vi "Write_Parameter_To_Node_Test.vi"() -> ()   [LabVIEW 2017]
uses:
  Classes/ADCP.lvclass
panel:
  in  "ADCP in":refnum<class "ADCP.lvclass">
  in  "Write Parameter":bool
  in  "Parameter value":string
  in  "Parameter name":string(combo)
  in  "Stop Application":bool
  in  "Symbol File Path":path
  in  "ADCP Session Parameters":T1={"Symbol File Path"=path "", "Transmit Log File Path"=path "", "Receive Log File Path"=path "", "COM Port"="COM13", "Baud rate"=0, "Number of retries"=0, "Retry interval (ms)"=0, "Session start time (ms)"=0, "Current time (ms)"=0, "Serialport timeout (ms)"=0}
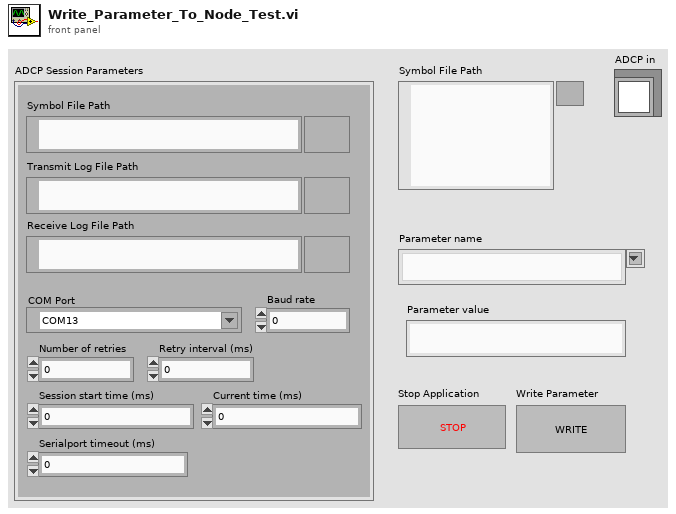
[diagram p1: front panel]
types:
  T1 = cluster{"Symbol File Path":path, "Transmit Log File Path":path, "Receive Log File Path":path, "COM Port":refnum<visa-resource-name>, "Baud rate":u32, "Number of retries":u16, "Retry interval (ms)":u16, "Session start time (ms)":u32, "Current time (ms)":u32, "Serialport timeout (ms)":u32}
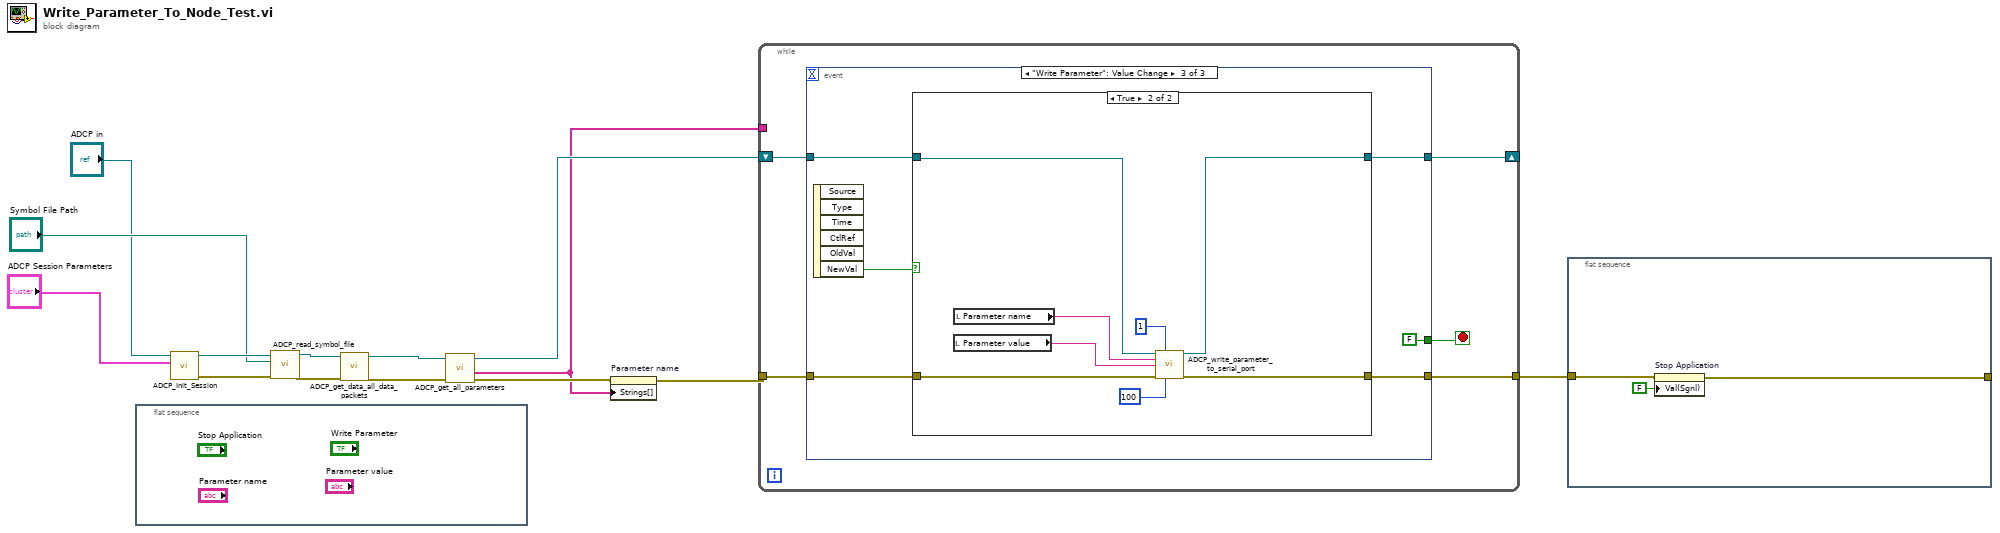
[diagram p0: block diagram]
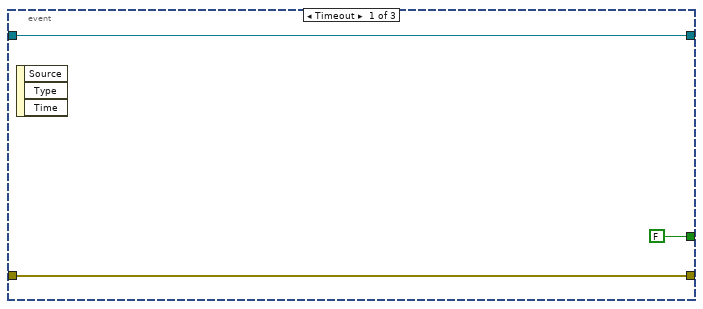
[diagram p2: hidden frame]
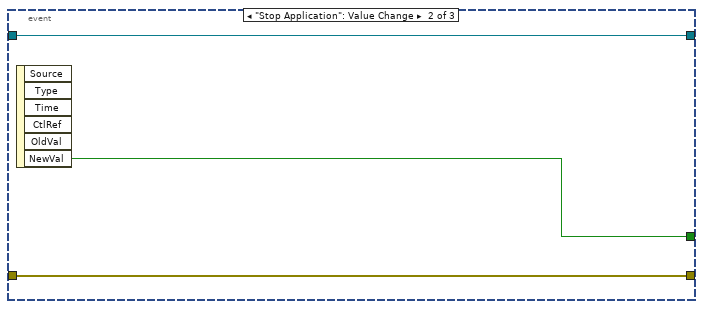
[diagram p3: hidden frame]
diagram:
  n1 = flat-sequence {
    frame #0 {
    }
  }
  n2 = call "ADCP_Init_Session.vi"("ADCP Session Parameters"="ADCP Session Parameters", "ADCP in"="ADCP in") -> ("error out"=w12:errorcluster, "ADCP out"=w13:refnum<class "ADCP.lvclass">)  [unwired: 8 in]
  n3 = call "ADCP_read_symbol_file.vi"("error in (no error)"=w12, "Symbol File Path"="Symbol File Path", "ADCP in"=w13) -> ("error out"=w9:errorcluster, "ADCP out"=w8:refnum<class "ADCP.lvclass">)  [unwired: 5 in, 2 out]
  n4 = call "ADCP_get_data_all_data_packets.vi"("error in (no error)"=w9, "ADCP In"=w8) -> ("error out"=w7:errorcluster, "ADCP Out"=w6:refnum<class "ADCP.lvclass">)  [unwired: 7 in, 1 out]
  n5 = call "ADCP_get_all_parameters.vi"("error in (no error)"=w7, "ADCP In"=w6) -> ("error out"=w4:errorcluster, "Parameter names"=w2:string[], "ADCP Out"=w5:refnum<class "ADCP.lvclass">)  [unwired: 6 in, 1 out]
  n6 = property on="Parameter name" class="CmbBox"(error in=w4, "Strings[]"=w2) -> (error out=w3:errorcluster)  [unwired: 1 in, 1 out]
  n7 = while {
    tunnel: w3 -> [w17]
    shift-right: [w18] -> _
    shift-left: w5 -> [w19]
    tunnel: [w16] -> w10
    tunnel: w2 -> [_]
    stop <- w15 stop-if-true
    n8 = event shown="[2] \"Write Parameter\": Value Change" {
      selector: _ -> [_ _ _]
      dyn-events: _ -> [_ _ _]
      timeout: _ -> [_ _ _]
      tunnel: w19 -> [w22 w25 w29]
      tunnel: [w22 w25 w28] -> w18
      tunnel: w17 -> [w21 w23 w30]
      tunnel: [w21 w23 w27] -> w16
      tunnel: [FALSE w24 FALSE ("NewVal")] -> w15
      event Timeout {
        n9 = event-data() -> ()  [unwired: 1 in, 3 out]
      }
      event "Stop Application": Value Change {
        n10 = event-data() -> ("NewVal"=w24:bool)  [unwired: 1 in, 5 out]
      }
      event "Write Parameter": Value Change {
        n11 = event-data() -> ("NewVal"=w26:bool)  [unwired: 1 in, 5 out]
        n12 = case shown="True" w26 {
          tunnel: w30 -> [w32 w41]
          tunnel: w29 -> [w33 w37]
          tunnel: [w33 w36] -> w28
          tunnel: [w32 w40] -> w27
          frame False {
          }
          frame True {
            n13 = local read "Parameter value"() -> (w34:string)
            n14 = local read "Parameter name"() -> (w35:string)
            n15 = call "ADCP_write_parameter_to_serial_port.vi"("ADCP In"=w37, "Transmit count"=u32 1, "Parameter name"=w35, "Parameter value"=w34, "error in (no error)"=w41, "Transmit interval (ms)"=u32 100) -> ("ADCP out"=w36:refnum<class "ADCP.lvclass">, "error out"=w40:errorcluster)  [unwired: 6 in, 2 out]
          }
        }
      }
    }
  }
  n16 = flat-sequence {
    tunnel: w10 -> [w44]
    tunnel: [w43] -> _
    frame #0 {
      n17 = property on="Stop Application" class="Bool (strict)"(error in=w44, "Val(Sgnl)"=FALSE ("Value (Signaling)")) -> (error out=w43:errorcluster)  [unwired: 1 in, 1 out]
    }
  }
